vi "VI Server_Get Combo Box Values_SpreadSheetStr.vi"(7 "Label":string, 8 "error in":errorcluster, 9 "Single Instance (T)":bool=TRUE, 11 "VI Server Cluster":T1) -> (0 "error out":errorcluster, 1 "Control Reference":refnum<vi>, 2 "Values.Spreadsheet STR":string caption="Strings [].Spreadsheet STR", 3 "VI Server Custer.DUP":T1={"Labels"=["Label", "Size", "Font", "Heght", "Width", "Ledding Denominator", "Ledding Nominator", "Label Number", "Microstep Resolution", "X", "Y", "Z", "Italic?", "Underlined?"], "Refs"=[], "VI Ref"=refnum}, 6 "Label.Text DUP":string)   [LabVIEW 2020, in "VI Server Toolkit LV2013.lvlib"]
doc: "Returns item names (STR array) of the Text Ring converted into a spreadsheet string.\n\nUsed for saving the text ring contents into configuration file."
uses:
  VI Server Toolkit LV2013.lvlib
  VI Server_TypeDefs/VI Server_RefsCluster.ctl
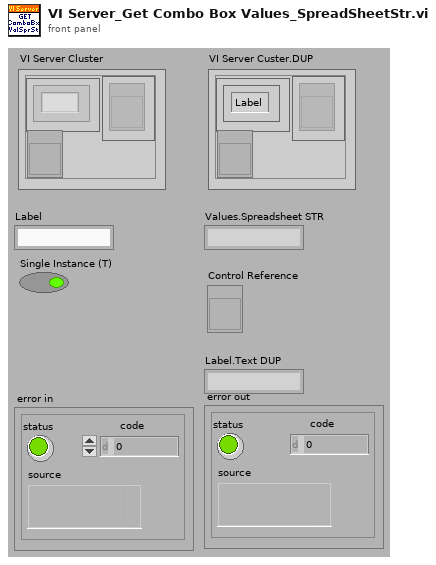
[diagram p1: front panel]
types:
  T1 = typedef "VI Server_RefsCluster.ctl" = cluster{"Labels":string[], "Refs":refnum<vi>[], "VI Ref":refnum<vi>}
  T2 = typedef "LVComboBoxStrsAndValuesArrayTypeDef.ctl" = cluster{"String":string, "Value":string}[]
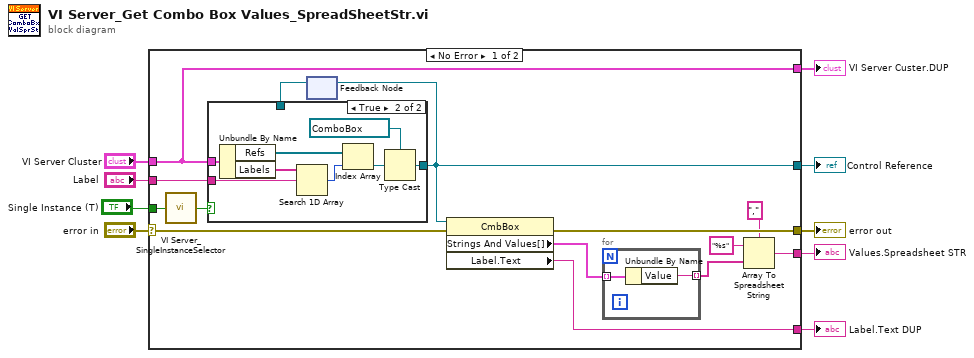
[diagram p0: block diagram]
diagram:
  n1 = case shown="No Error" "error in" {
    selector: "error in" -> [w22 w35]
    tunnel: "Label" -> [w23 _]
    tunnel: "VI Server Cluster" -> [w19 _]
    tunnel: [w21 w35] -> w9
    tunnel: [w13 _] -> w1
    tunnel: [w20 _] -> w5
    tunnel: [w19 _] -> w4
    tunnel: [w16 _] -> w3
    tunnel: "Single Instance (T)" -> [w14 _]
    frame No Error {
      n2 = call "VI Server_SingleInstanceSelector.vi"("Single Instance (T)"=w14) -> ("Single Instance.OUT"=w15:bool)  [unwired: 6 in]
      n3 = feedback #1() -> (w12:refnum<vi>)  [unwired: 1 in]
      n4 = case shown="True" w15 {
        tunnel: w23 -> [_ w33]
        tunnel: [w26 w29] -> w13
        tunnel: w19 -> [_ w28]
        tunnel: w12 -> [w26 _]
        frame False {
        }
        frame True {
          n5 = Unbundle By Name(w28) -> ("Refs"=w31:refnum<vi>[], "Labels"=w34:string[])
          n6 = Search 1D Array(1D array=w34, element=w33) -> (index of element=w32:i32)  [unwired: 1 out]
          n7 = Index Array(array=w31, index=w32) -> (element=w30:refnum<vi>)
          n8 = Type Cast(type=refnum<vi> refnum ("OS.SelectChannel"), x=w30) -> (*(type *) &x=w29:refnum<vi>)
        }
      }
      n9 = feedback-in #1(w13) -> ()
      n10 = property class="CmbBox"(reference=w13, error in=w22) -> (error out=w21:errorcluster, "Strings And Values[]"=w11:T2, "Label.Text"=w20:string)  [unwired: 1 out]
      n11 = for {
        tunnel: w11 -> [w25] mode=indexing
        tunnel: [w24] -> w10 mode=indexing
        n12 = Unbundle By Name(w25) -> ("Value"=w24:string)
      }
      n13 = Array To Spreadsheet String(delimiter (Tab)=",", array=w10, 3:"%s" ("format string")) -> (spreadsheet string=w16:string)
    }
    frame Error {
    }
  }
  "error out" <- w9
  "VI Server Custer.DUP" <- w4
  "Label.Text DUP" <- w5
  "Values.Spreadsheet STR" <- w3
  "Control Reference" <- w1
